vi "HEWH MW100 Cut Unneeded Raw Data.vi"(10 "MW100 Data In":string[][](array[string])) -> (2 "MW100 Data Out":string[][](array[string]))   [LabVIEW 2012]
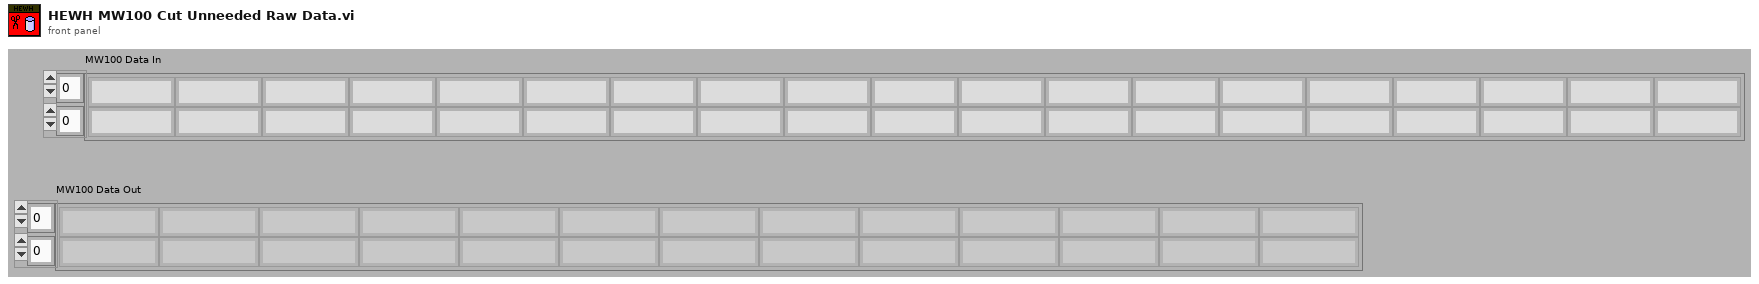
[diagram p1: front panel]
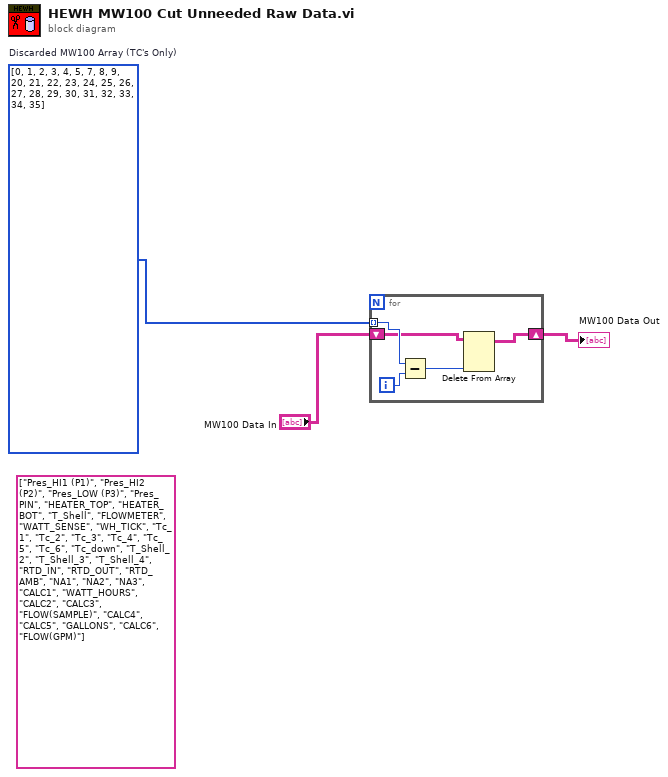
[diagram p0: block diagram]
diagram:
  w1 = i32[] [0, 1, 2, 3, 4, 5, 7, 8, 9, 20, 21, 22, 23, 24, 25, 26, 27, 28, 29, 30, 31, 32, 33, 34, 35]  # Discarded MW100 Array (TC's Only)
  (unwired) string[] ["Pres_HI1 (P1)", "Pres_HI2 (P2)", "Pres_LOW (P3)", "Pres_PIN", "HEATER_TOP", "HEATER_BOT", "T_Shell", "FLOWMETER", "WATT_SENSE", "WH_TICK", "Tc_1", "Tc_2", "Tc_3", "Tc_4", "Tc_5", "Tc_6", "Tc_down", "T_Shell_2", "T_Shell_3", "T_Shell_4", "RTD_IN", "RTD_OUT", "RTD_AMB", "NA1", "NA2", "NA3", "CALC1", "WATT_HOURS", "CALC2", "CALC3", "FLOW(SAMPLE)", "CALC4", "CALC5", "GALLONS", "CALC6", "FLOW(GPM)"] ("output array")
  n1 = for {
    tunnel: w1 -> [w7] mode=indexing
    shift-right: [w5] -> w3
    shift-left: "MW100 Data In" -> [w4]
    i -> [w8]
    n2 = Subtract(x=w7, y=w8) -> (x-y=w6:i32)
    n3 = Delete From Array(array=w4, index (col)=w6) -> (array with subset deleted=w5:string[][])  [unwired: 2 in, 1 out]
  }
  "MW100 Data Out" <- w3
